vi "LPG.vi"() -> ()   [LabVIEW 2019]
uses:
  <vilib>/MakerHub/LINX/Public/Peripherals/Analog/Analog Read 1 Chan.vi
  <vilib>/MakerHub/LINX/Public/Peripherals/Analog/Analog Read N Chans.vi
  <vilib>/MakerHub/LINX/Private/Local IO/LinxAnalogRead.vi
  <vilib>/MakerHub/LINX/Public/Utilities/Check Channel.vi
  <vilib>/MakerHub/LINX/Public/Utilities/Open Serial.vi
  <vilib>/MakerHub/LINX/Private/Utilties/Generate Error.vi
  <vilib>/MakerHub/LINX/Public/Sensors/Motion/Servo/Servo Open One Channel.vi
  <vilib>/MakerHub/LINX/Public/Sensors/Motion/Servo/Servo Set Pulse Width One Channel.vi
  <vilib>/MakerHub/LINX/Public/Sensors/Motion/Servo/Servo Close One Channel.vi
  <vilib>/MakerHub/LINX/LMH-LINX.lvlib
  <vilib>/MakerHub/LINX/Public/Sensors/Motion/Servo/Servo.lvlib
  <vilib>/Analysis/NI_AALPro.lvlib
panel:
  out "servo angle":i32
  out "THREAT":bool
  out "concentration":dbl
  out "avg read":dbl
  out "r":dbl
  out "calib avg":dbl
  out "read Voltage":dbl
  out "loop 2":i32
  out "loop1":i32
  out "r0":dbl
  out "concentration chart":dbl(graph)
  in  "gas sensor pin":u8
  out "calib Voltage":dbl
  in  "stop":bool
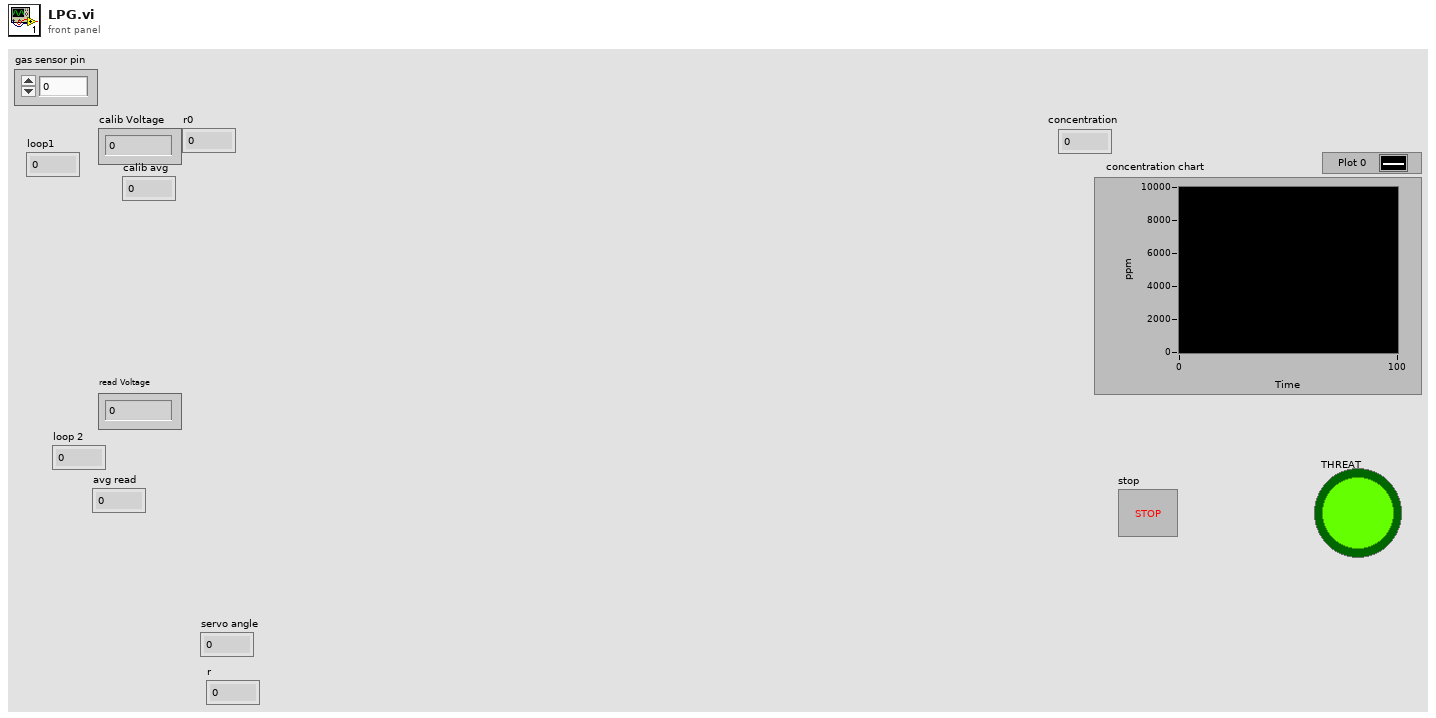
[diagram p1: front panel]
types:
  T1 = typedef "LMH-LINX.lvlib/LINX Ref.ctl" = cluster{"IO":T2, "Interface":T3, "LINX Device Config":T4}
  T2 = typedef "LMH-LINX.lvlib/Platform.ctl" = enum16{"Remote", "Local"}
  T3 = typedef "LMH-LINX.lvlib/Interface.ctl" = enum16{"Serial", "TCP"}
  T4 = typedef "LMH-LINX.lvlib/Device.lvlib/LINX Device Config.ctl" = cluster{"Interface":T3, "COM Port":refnum<visa-resource-name>, "TCP Configuration":T5, "Device Family":u8, "Device ID":u8, "Device Name":string, "TCP Ref":refnum<k5>, "Channels":T6}
  T5 = typedef "LMH-LINX.lvlib/Device.lvlib/TCP Config.ctl" = cluster{"IP Address":string, "Port":u16}
  T6 = typedef "LMH-LINX.lvlib/Channels.ctl" = cluster{"DI":u8[], "DO":u8[], "AI":u8[], "AO":u8[], "PWM":u8[], "QE":u8[], "UART":u8[], "I2C 2":u8[], "SPI":u8[], "CAN":u8[], "Servo":u8[], "AI Ref (V)":dbl, "AI Resolution (Bits)":u8, "AO Ref (V)":dbl, "AO Resolution (Bits)":u8}
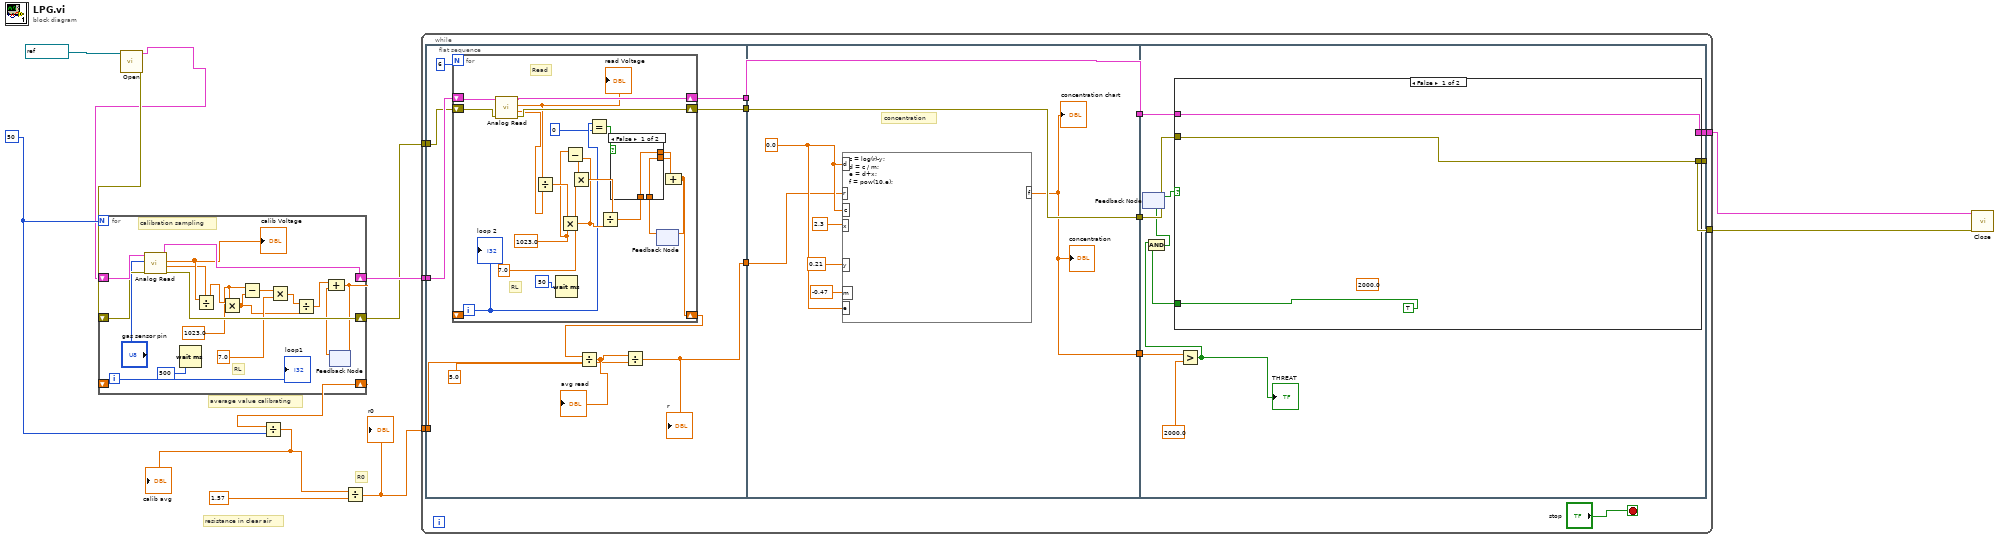
[diagram p0: block diagram]
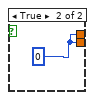
[diagram p2: hidden frame]
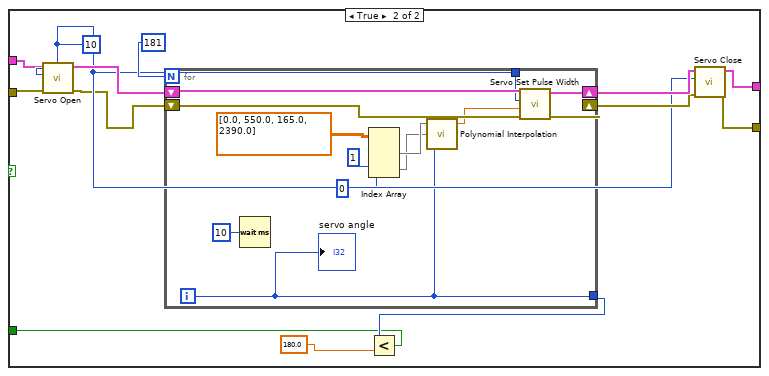
[diagram p3: hidden frame]
diagram:
  w12 = 50
  # "R0"
  # "resistance in clear air"
  # "average value calibrating"
  n1 = call-poly <vilib>:"Open.vi"("Serial Port"=refnum<visa-resource-name> "COM3") -> ("Error Out"=w5:errorcluster, "LINX Resource"=w4:T1)  [unwired: 8 in, 1 out]
  n2 = for {
    N: w12 -> [_]
    shift-right: [w28] -> w7
    shift-left: w4 -> [w30]
    shift-right: [w27] -> w6
    shift-left: w5 -> [w29]
    shift-right: [w24] -> w11
    shift-left: _ -> [_]
    i -> [w13]
    w19 = 1023.0 ("y")
    # "RL"
    # "calibration sampling"
    n3 = call-poly <vilib>:"Analog Read.vi"("Error In"=w29, "Analog Channel"="gas sensor pin", "LINX Resource"=w30) -> ("Error Out"=w27:errorcluster, "AI Ref"=w21:dbl, "Voltage"=w22:dbl, "LINX Resource"=w28:T1)  [unwired: 5 in]
    "calib Voltage" <- w22
    n4 = Wait (ms)(milliseconds to wait=u32 500) -> ()  [unwired: 1 out]
    n5 = Divide(x=w22, y=w21) -> (x/y=w20:dbl)
    n6 = Multiply(x=w20, y=w19) -> (x*y=w15:dbl)
    n7 = Subtract(x=w19, y=w15) -> (x-y=w18:dbl)
    n8 = Multiply(x=w18, y=7.0) -> (x*y=w16:dbl)
    n9 = Divide(x=w16, y=w15) -> (x/y=w14:dbl)
    n10 = feedback #1() -> (w26:dbl)  [unwired: 1 in]
    n11 = Compound Arithmetic op=ADD(w14, w26) -> (w24:dbl)
    n12 = feedback-in #1(w24) -> ()
    "loop1" <- w13
  }
  n13 = Divide(x=w11, y=w12) -> (x/y=w10:dbl)
  "calib avg" <- w10
  n14 = Divide(x=w10, y=1.57) -> (x/y=w8:dbl)
  "r0" <- w8
  n15 = while {
    tunnel: w8 -> [w31]
    tunnel: w7 -> [w42]
    tunnel: w6 -> [w41]
    tunnel: [w38] -> w3
    tunnel: [w35] -> w2
    stop <- "stop" stop-if-true
    n16 = flat-sequence {
      tunnel: w42 -> [w52]
      tunnel: w41 -> [w51]
      tunnel: [w50] -> w39
      tunnel: [w49] -> w36
      tunnel: [w43] -> w32
      tunnel: w31 -> [w44]
      tunnel: [w79] -> w40
      tunnel: w39 -> [w79]
      tunnel: [w78] -> w37
      tunnel: w36 -> [w78]
      tunnel: [w77] -> w34
      tunnel: w32 -> [w80]
      tunnel: w40 -> [w94]
      tunnel: [w93] -> w38
      tunnel: w37 -> [w91]
      tunnel: [w92] -> w35
      tunnel: w34 -> [w89]
      frame #0 {
        n17 = for {
          N: 6 -> [_]
          shift-right: [w69] -> w49
          shift-left: w51 -> [w71]
          shift-right: [w70] -> w50
          shift-left: w52 -> [w72]
          shift-right: [w60] -> w48
          shift-left: _ -> [_]
          i -> [w54]
          w65 = 1023.0 ("y")
          # "Read"
          # "RL"
          n18 = call-poly <vilib>:"Analog Read.vi"("Error In"=w71, "LINX Resource"=w72) -> ("Error Out"=w69:errorcluster, "AI Ref"=w67:dbl, "Voltage"=w68:dbl, "LINX Resource"=w70:T1)  [unwired: 6 in]
          "read Voltage" <- w68
          n19 = Divide(x=w68, y=w67) -> (x/y=w66:dbl)
          n20 = Wait (ms)(milliseconds to wait=u32 50) -> ()  [unwired: 1 out]
          n21 = Multiply(x=w66, y=w65) -> (x*y=w61:dbl)
          n22 = Subtract(x=w65, y=w61) -> (x-y=w64:dbl)
          n23 = Multiply(x=w64, y=7.0) -> (x*y=w62:dbl)
          n24 = Equal?(x=w54, y=0) -> (x = y?=w55:bool)
          n25 = Divide(x=w62, y=w61) -> (x/y=w58:dbl)
          n26 = feedback #2() -> (w57:dbl)  [unwired: 1 in]
          n27 = case shown="False" w55 {
            tunnel: [w75 w76] -> w59
            tunnel: w58 -> [w75 _]
            tunnel: w57 -> [w74 _]
            tunnel: [w74 w76] -> w56
            frame False {
            }
            frame True {
              w76 = 0
            }
          }
          n28 = Compound Arithmetic op=ADD(w59, w56) -> (w60:dbl)
          n29 = feedback-in #2(w60) -> ()
          "loop 2" <- w54
        }
        n30 = Divide(x=w48, y=5.0) -> (x/y=w45:dbl)
        "avg read" <- w45
        n31 = Divide(x=w44, y=w45) -> (x/y=w43:dbl)
        "r" <- w43
      }
      frame #1 {
        w81 = 0.0 ("input variable")
        # "concentration"
        n32 = formula code="c = log(r)-y;\nd = c / m;\ne = d+x;\nf = pow(10,e);"("r"=w80, "y"=0.21 ("input variable"), "m"=-0.47 ("input variable"), "x"=2.3 ("input variable"), "d"=w81, "e"=w81, "c"=w81) -> ("f"=w77:dbl)
        "concentration chart" <- w77
        "concentration" <- w77
      }
      frame #2 {
        (unwired) 2000.0 ("y")
        n33 = feedback #3() -> (w86:bool)  [unwired: 1 in]
        n34 = case shown="False" w86 {
          tunnel: [w96 w103] -> w92
          tunnel: [w97 w104] -> w93
          tunnel: w94 -> [w97 w105]
          tunnel: w91 -> [w96 w99]
          tunnel: [TRUE w101] -> w85
          frame False {
          }
          frame True {
            w106 = u8 10 ("Servo Channel")
            n35 = call-poly <vilib>:"Servo Open.vi"("Error In"=w99, "Servo Channel"=w106, "LINX Resource"=w105) -> ("Error Out"=w98:errorcluster, "LINX Resource"=w109:T1)  [unwired: 7 in]
            n36 = for {
              N: 181 -> [_]
              tunnel: w106 -> [w119]
              shift-right: [w122] -> w108
              shift-left: w109 -> [w123]
              shift-right: [w120] -> w107
              shift-left: w98 -> [w121]
              tunnel: [w111] -> w102
              i -> [w111]
              n37 = Wait (ms)(milliseconds to wait=u32 10) -> ()  [unwired: 1 out]
              n38 = Index Array(array=dbl[][] [[0.0, 550.0], [165.0, 2390.0]], index (col) #1=1 ("disabled index (col)"), index (col) #2=0 ("index (col)")) -> (element #1=w114:dbl[], element #2=w113:dbl[])  [unwired: 2 in]
              n39 = call <vilib>:"Polynomial Interpolation.vi"("x value"=w111, "X"=w113, "Y"=w114) -> ("interpolation value"=w118:dbl)  [unwired: 2 out]
              n40 = call-poly <vilib>:"Servo Set Pulse Width.vi"("Error In"=w121, "Pulse Width (uS)"=w118, "Servo Channel"=w119, "LINX Resource"=w123) -> ("Error Out"=w120:errorcluster, "LINX Resource"=w122:T1)  [unwired: 6 in]
              "servo angle" <- w111
            }
            n41 = Less?(x=w102, y=180.0) -> (x < y?=w101:bool)
            n42 = call-poly <vilib>:"Servo Close.vi"("Error In"=w107, "Servo Channel"=w106, "LINX Resource"=w108) -> ("Error Out"=w103:errorcluster, "LINX Resource"=w104:T1)  [unwired: 7 in]
          }
        }
        n43 = Greater?(x=w89, y=2000.0) -> (0:w88:bool)
        "THREAT" <- w88
        n44 = And(x=w88, y=w85) -> (x .and. y?=w87:bool)
        n45 = feedback-in #3(w87) -> ()
      }
    }
  }
  n46 = call <vilib>:"Close.vi"("Error In"=w2, "LINX Resource"=w3) -> ()  [unwired: 9 in, 1 out]
